vi "Mem_LvDataToMemory_NOPTR.vi"(8 "error in (no error)":errorcluster, 10 "Payload":variant) -> (0 "error out":errorcluster, 1 "Supported Type?":bool, 2 "ByteArray":u8[](array[numeric]))   [LabVIEW 2019, in "Memory Data Access.lvlib"]
uses:
  Memory Data Access.lvlib
  <vilib>/Utility/Data Type/Type Definitions/Data Type.ctl
  Global/Global.vi
  <vilib>/Utility/Data Type/NI_Data Type.lvlib
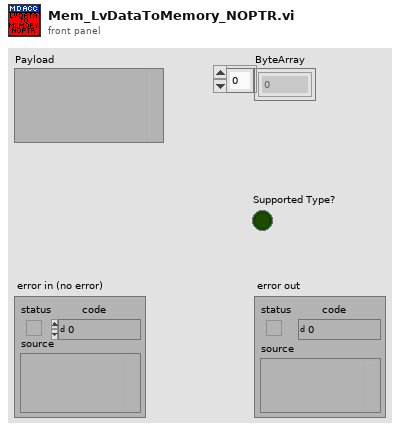
[diagram p1: front panel]
types:
  T1 = typedef "NI_Data Type.lvlib/Data Type.ctl" = enum8{"Invalid Type", "Void", "I8", "I16", "I32", "I64", "U8", "U16", "U32", "U64", "Single Float", "Double Float", "Extended Float", "Single Complex", "Double Complex", "Extended Complex", "Enum U8", "Enum U16", "Enum U32", "Enum U64", "Single Float With Unit", "Double Float With Unit", "Extended Float With Unit", "Single Complex with Unit", "Double Complex with Unit", "Extended Complex with Unit", "Boolean", "String", "Path", "Picture", "Tag", "Array", "Cluster", "Variant", "LV Variant", "Waveform", "Timestamp", "Digital Waveform", "Digital Data", "ExpressData", "Refnum", "External Data", "VI", "Poly VI", "LabVIEW Class Instance", "Fixed Point", "Set Collection", "Map Collection"}
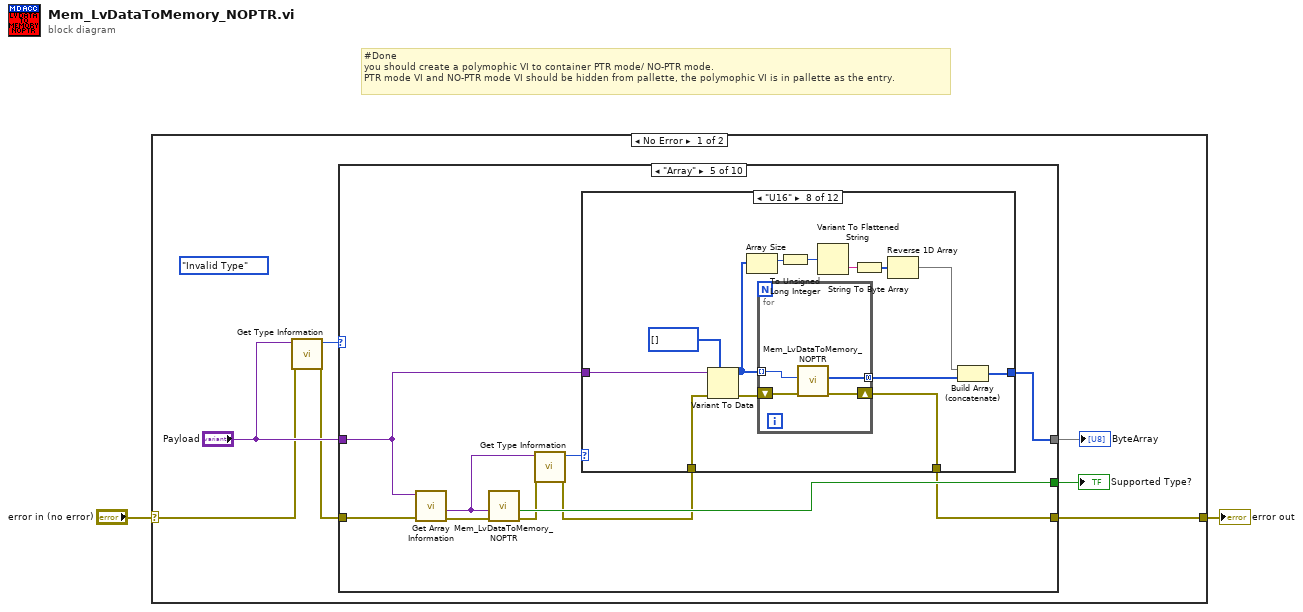
[diagram p0: block diagram]
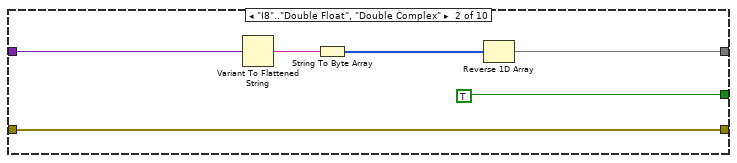
[diagram p3: hidden frame]
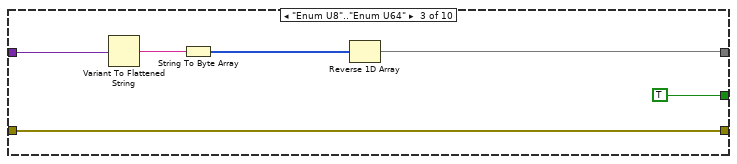
[diagram p4: hidden frame]
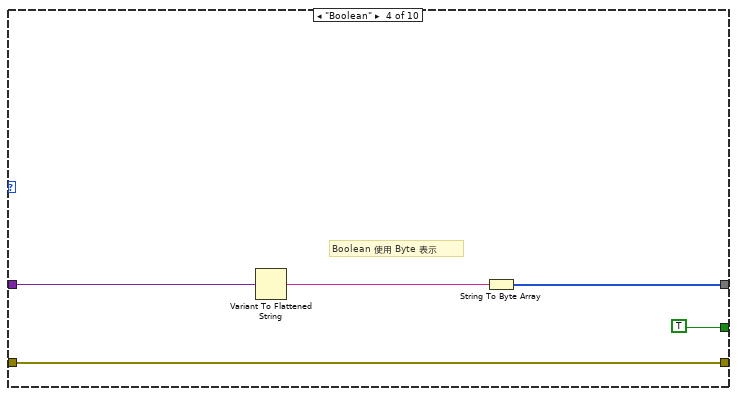
[diagram p5: hidden frame]
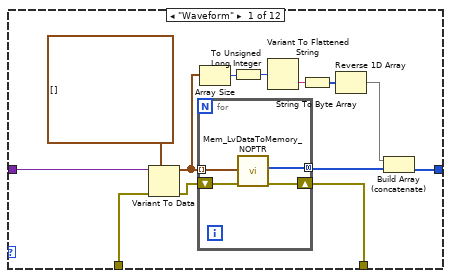
[diagram p6: hidden frame]
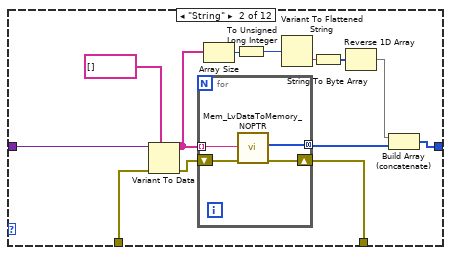
[diagram p7: hidden frame]
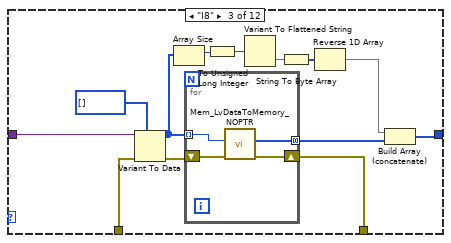
[diagram p8: hidden frame]
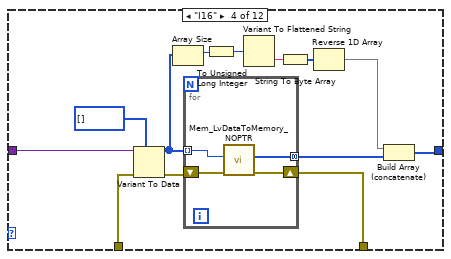
[diagram p9: hidden frame]
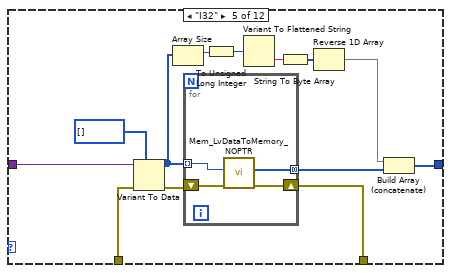
[diagram p10: hidden frame]
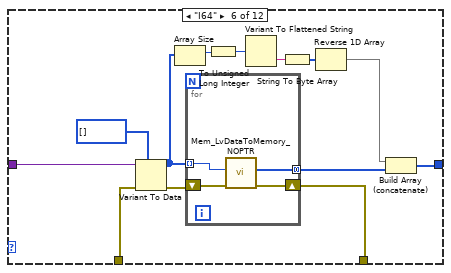
[diagram p11: hidden frame]
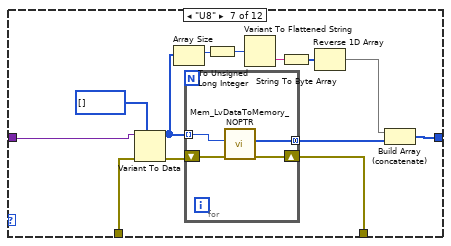
[diagram p12: hidden frame]
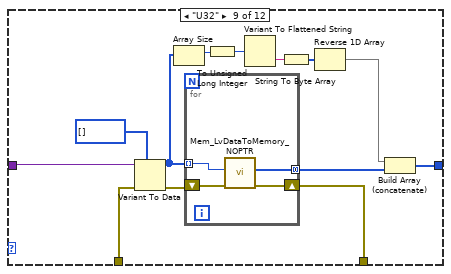
[diagram p13: hidden frame]
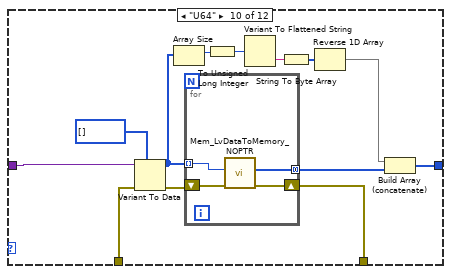
[diagram p14: hidden frame]
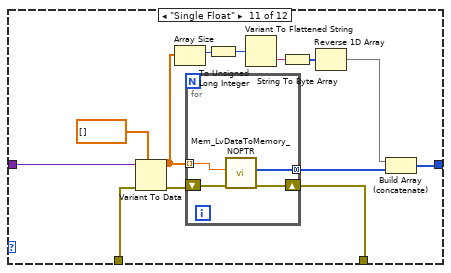
[diagram p15: hidden frame]
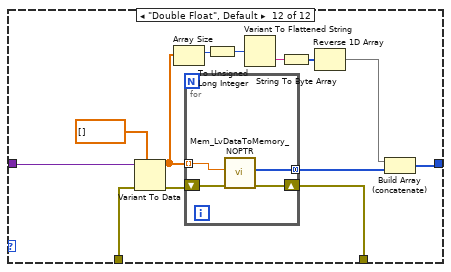
[diagram p16: hidden frame]
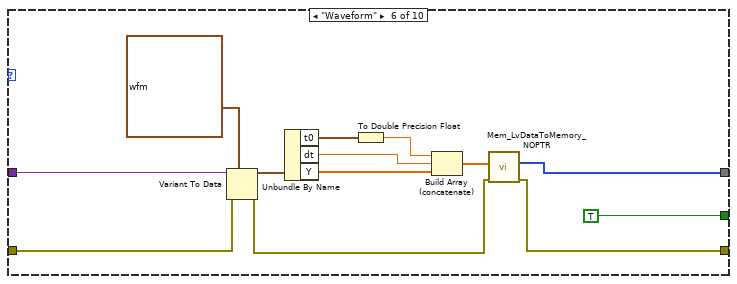
[diagram p17: hidden frame]
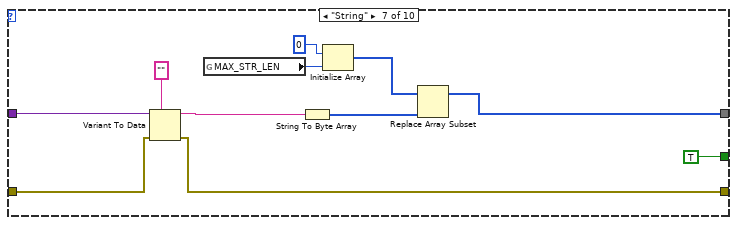
[diagram p18: hidden frame]
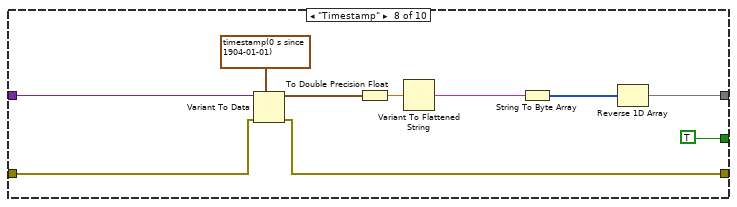
[diagram p19: hidden frame]
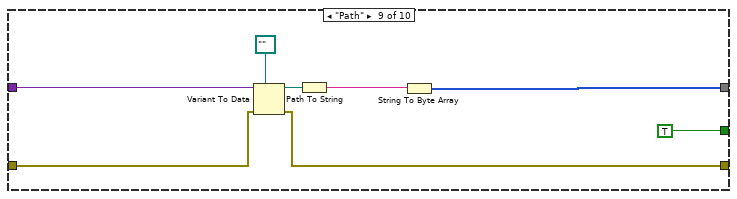
[diagram p20: hidden frame]
diagram:
  # "#Done\nyou should create a polymophic VI to container PTR mode/ NO-PTR mode.\nPTR mode VI and NO-PTR mode VI should be hidden from pallette, the polymophic VI is in pallette as the entry."
  n1 = case shown="No Error" "error in (no error)" {
    selector: "error in (no error)" -> [w4 w298]
    tunnel: [w9 w298] -> w2
    frame No Error {
      (unwired) Data_Type."Invalid Type" ("Type")
      n2 = call <vilib>:"Get Type Information.vi"("error in (no error)"=w4, "variant"="Payload") -> ("error out"=w3:errorcluster, "type"=w5:T1)  [unwired: 5 in, 3 out]
      n3 = case shown="\"Array\"" w5 {
        tunnel: w3 -> [w10 w16 w18 w27 w33 w246 w260 w270 w278 w284]
        tunnel: [w10 w16 w18 w27 w35 w243 w261 w271 w279 w285] -> w9
        tunnel: [_ w11 w19 w23 w37 w242 w263 w266 w281 w289] -> w8
        tunnel: "Payload" -> [_ w14 w21 w25 w34 w253 w264 w274 w282 w292]
        tunnel: [_ TRUE TRUE ("Supported Type?") TRUE w36 TRUE TRUE TRUE TRUE w287] -> w7
        frame "Invalid Type", Default {
        }
        frame "I8".."Double Float", "Double Complex" {
          n4 = Variant To Flattened String(Variant=w14) -> (data string=w13:string)  [unwired: 1 out]
          n5 = String To Byte Array(string=w13) -> (unsigned byte array=w12:u8[])
          n6 = Reverse 1D Array(array=w12) -> (reversed array=w11:u8[])
        }
        frame "Enum U8".."Enum U64" {
          n7 = Variant To Flattened String(Variant=w21) -> (data string=w22:string)  [unwired: 1 out]
          n8 = String To Byte Array(string=w22) -> (unsigned byte array=w20:u8[])
          n9 = Reverse 1D Array(array=w20) -> (reversed array=w19:u8[])
        }
        frame "Boolean" {
          # "Boolean 使用 Byte 表示"
          n10 = Variant To Flattened String(Variant=w25) -> (data string=w24:string)  [unwired: 1 out]
          n11 = String To Byte Array(string=w24) -> (unsigned byte array=w23:u8[])
        }
        frame "Array" {
          n12 = call <vilib>:"Get Array Information.vi"("error in (no error)"=w33, "variant"=w34) -> ("error out"=w32:errorcluster, "array element data type"=w30:variant)  [unwired: 6 in, 2 out]
          n13 = call "Mem_LvDataToMemory_NOPTR.vi"("error in (no error)"=w32, "Payload"=w30) -> ("error out"=w29:errorcluster, "Supported Type?"=w36:bool)  [unwired: 7 in, 1 out]
          n14 = call <vilib>:"Get Type Information.vi"("error in (no error)"=w29, "variant"=w30) -> ("error out"=w28:errorcluster, "type"=w31:T1)  [unwired: 5 in, 3 out]
          n15 = case shown="\"U16\"" w31 {
            tunnel: [w47 w64 w73 w90 w107 w124 w144 w161 w178 w195 w211 w226] -> w37
            tunnel: w34 -> [w50 w67 w83 w91 w110 w127 w143 w160 w177 w194 w212 w229]
            tunnel: w28 -> [w45 w62 w84 w93 w109 w126 w142 w159 w176 w193 w210 w228]
            tunnel: [w44 w61 w74 w92 w108 w125 w141 w158 w175 w192 w209 w227] -> w35
            frame "Waveform" {
              n16 = Variant To Data(error in=w45, type=waveform(dbl)[] [] ("Waveform"), Variant=w50) -> (data=w43:waveform(dbl)[], error out=w46:errorcluster)
              n17 = for {
                tunnel: w43 -> [w54] mode=indexing
                tunnel: [w53] -> w48 mode=concatenating
                shift-right: [w51] -> w44
                shift-left: w46 -> [w52]
                n18 = call "Mem_LvDataToMemory_NOPTR.vi"("error in (no error)"=w52, "Payload"=w54) -> ("error out"=w51:errorcluster, "ByteArray"=w53:u8[])  [unwired: 7 in, 1 out]
              }
              n19 = Array Size(array=w43) -> (size(s)=w42:i32)
              n20 = To Unsigned Long Integer(number=w42) -> (unsigned 32bit integer=w40:u32)
              n21 = Variant To Flattened String(Variant=w40) -> (data string=w41:string)  [unwired: 1 out]
              n22 = String To Byte Array(string=w41) -> (unsigned byte array=w39:u8[])
              n23 = Reverse 1D Array(array=w39) -> (reversed array=w38:u8[])
              n24 = Build Array (concatenate)(w38, w48) -> (w47:u8[])
            }
            frame "String" {
              n25 = Variant To Data(error in=w62, type=string[] [] ("Waveform"), Variant=w67) -> (data=w60:string[], error out=w63:errorcluster)
              n26 = for {
                tunnel: w60 -> [w71] mode=indexing
                tunnel: [w70] -> w65 mode=concatenating
                shift-right: [w68] -> w61
                shift-left: w63 -> [w69]
                n27 = call "Mem_LvDataToMemory_NOPTR.vi"("error in (no error)"=w69, "Payload"=w71) -> ("error out"=w68:errorcluster, "ByteArray"=w70:u8[])  [unwired: 7 in, 1 out]
              }
              n28 = Array Size(array=w60) -> (size(s)=w59:i32)
              n29 = To Unsigned Long Integer(number=w59) -> (unsigned 32bit integer=w57:u32)
              n30 = Variant To Flattened String(Variant=w57) -> (data string=w58:string)  [unwired: 1 out]
              n31 = String To Byte Array(string=w58) -> (unsigned byte array=w56:u8[])
              n32 = Reverse 1D Array(array=w56) -> (reversed array=w55:u8[])
              n33 = Build Array (concatenate)(w55, w65) -> (w64:u8[])
            }
            frame "I8" {
              n34 = Variant To Data(error in=w84, type=i8[] [], Variant=w83) -> (data=w72:i8[], error out=w82:errorcluster)
              n35 = Array Size(array=w72) -> (size(s)=w78:i32)
              n36 = for {
                tunnel: [w88] -> w75 mode=concatenating
                shift-right: [w86] -> w74
                shift-left: w82 -> [w87]
                tunnel: w72 -> [w85] mode=indexing
                n37 = call "Mem_LvDataToMemory_NOPTR.vi"("error in (no error)"=w87, "Payload"=w85) -> ("error out"=w86:errorcluster, "ByteArray"=w88:u8[])  [unwired: 7 in, 1 out]
              }
              n38 = To Unsigned Long Integer(number=w78) -> (unsigned 32bit integer=w79:u32)
              n39 = Variant To Flattened String(Variant=w79) -> (data string=w80:string)  [unwired: 1 out]
              n40 = String To Byte Array(string=w80) -> (unsigned byte array=w77:u8[])
              n41 = Reverse 1D Array(array=w77) -> (reversed array=w76:u8[])
              n42 = Build Array (concatenate)(w76, w75) -> (w73:u8[])
            }
            frame "I16" {
              n43 = Variant To Data(error in=w93, type=i16[] [], Variant=w91) -> (data=w89:i16[], error out=w101:errorcluster)
              n44 = Array Size(array=w89) -> (size(s)=w97:i32)
              n45 = for {
                tunnel: [w105] -> w94 mode=concatenating
                shift-right: [w103] -> w92
                shift-left: w101 -> [w104]
                tunnel: w89 -> [w102] mode=indexing
                n46 = call "Mem_LvDataToMemory_NOPTR.vi"("error in (no error)"=w104, "Payload"=w102) -> ("error out"=w103:errorcluster, "ByteArray"=w105:u8[])  [unwired: 7 in, 1 out]
              }
              n47 = To Unsigned Long Integer(number=w97) -> (unsigned 32bit integer=w98:u32)
              n48 = Variant To Flattened String(Variant=w98) -> (data string=w99:string)  [unwired: 1 out]
              n49 = String To Byte Array(string=w99) -> (unsigned byte array=w96:u8[])
              n50 = Reverse 1D Array(array=w96) -> (reversed array=w95:u8[])
              n51 = Build Array (concatenate)(w95, w94) -> (w90:u8[])
            }
            frame "I32" {
              n52 = Variant To Data(error in=w109, type=i32[] [], Variant=w110) -> (data=w106:i32[], error out=w118:errorcluster)
              n53 = Array Size(array=w106) -> (size(s)=w114:i32)
              n54 = for {
                tunnel: [w122] -> w111 mode=concatenating
                shift-right: [w120] -> w108
                shift-left: w118 -> [w121]
                tunnel: w106 -> [w119] mode=indexing
                n55 = call "Mem_LvDataToMemory_NOPTR.vi"("error in (no error)"=w121, "Payload"=w119) -> ("error out"=w120:errorcluster, "ByteArray"=w122:u8[])  [unwired: 7 in, 1 out]
              }
              n56 = To Unsigned Long Integer(number=w114) -> (unsigned 32bit integer=w115:u32)
              n57 = Variant To Flattened String(Variant=w115) -> (data string=w116:string)  [unwired: 1 out]
              n58 = String To Byte Array(string=w116) -> (unsigned byte array=w113:u8[])
              n59 = Reverse 1D Array(array=w113) -> (reversed array=w112:u8[])
              n60 = Build Array (concatenate)(w112, w111) -> (w107:u8[])
            }
            frame "I64" {
              n61 = Variant To Data(error in=w126, type=i64[] [], Variant=w127) -> (data=w123:i64[], error out=w135:errorcluster)
              n62 = Array Size(array=w123) -> (size(s)=w131:i32)
              n63 = for {
                tunnel: [w139] -> w128 mode=concatenating
                shift-right: [w137] -> w125
                shift-left: w135 -> [w138]
                tunnel: w123 -> [w136] mode=indexing
                n64 = call "Mem_LvDataToMemory_NOPTR.vi"("error in (no error)"=w138, "Payload"=w136) -> ("error out"=w137:errorcluster, "ByteArray"=w139:u8[])  [unwired: 7 in, 1 out]
              }
              n65 = To Unsigned Long Integer(number=w131) -> (unsigned 32bit integer=w132:u32)
              n66 = Variant To Flattened String(Variant=w132) -> (data string=w133:string)  [unwired: 1 out]
              n67 = String To Byte Array(string=w133) -> (unsigned byte array=w130:u8[])
              n68 = Reverse 1D Array(array=w130) -> (reversed array=w129:u8[])
              n69 = Build Array (concatenate)(w129, w128) -> (w124:u8[])
            }
            frame "U8" {
              n70 = Variant To Data(error in=w142, type=u8[] [], Variant=w143) -> (data=w140:u8[], error out=w152:errorcluster)
              n71 = Array Size(array=w140) -> (size(s)=w148:i32)
              n72 = for {
                tunnel: [w156] -> w145 mode=concatenating
                shift-right: [w154] -> w141
                shift-left: w152 -> [w155]
                tunnel: w140 -> [w153] mode=indexing
                n73 = call "Mem_LvDataToMemory_NOPTR.vi"("error in (no error)"=w155, "Payload"=w153) -> ("error out"=w154:errorcluster, "ByteArray"=w156:u8[])  [unwired: 7 in, 1 out]
              }
              n74 = To Unsigned Long Integer(number=w148) -> (unsigned 32bit integer=w149:u32)
              n75 = Variant To Flattened String(Variant=w149) -> (data string=w150:string)  [unwired: 1 out]
              n76 = String To Byte Array(string=w150) -> (unsigned byte array=w147:u8[])
              n77 = Reverse 1D Array(array=w147) -> (reversed array=w146:u8[])
              n78 = Build Array (concatenate)(w146, w145) -> (w144:u8[])
            }
            frame "U16" {
              n79 = Variant To Data(error in=w159, type=u16[] [], Variant=w160) -> (data=w157:u16[], error out=w169:errorcluster)
              n80 = Array Size(array=w157) -> (size(s)=w165:i32)
              n81 = for {
                tunnel: [w173] -> w162 mode=concatenating
                shift-right: [w171] -> w158
                shift-left: w169 -> [w172]
                tunnel: w157 -> [w170] mode=indexing
                n82 = call "Mem_LvDataToMemory_NOPTR.vi"("error in (no error)"=w172, "Payload"=w170) -> ("error out"=w171:errorcluster, "ByteArray"=w173:u8[])  [unwired: 7 in, 1 out]
              }
              n83 = To Unsigned Long Integer(number=w165) -> (unsigned 32bit integer=w166:u32)
              n84 = Variant To Flattened String(Variant=w166) -> (data string=w167:string)  [unwired: 1 out]
              n85 = String To Byte Array(string=w167) -> (unsigned byte array=w164:u8[])
              n86 = Reverse 1D Array(array=w164) -> (reversed array=w163:u8[])
              n87 = Build Array (concatenate)(w163, w162) -> (w161:u8[])
            }
            frame "U32" {
              n88 = Variant To Data(error in=w176, type=u32[] [], Variant=w177) -> (data=w174:u32[], error out=w186:errorcluster)
              n89 = Array Size(array=w174) -> (size(s)=w182:i32)
              n90 = for {
                tunnel: [w190] -> w179 mode=concatenating
                shift-right: [w188] -> w175
                shift-left: w186 -> [w189]
                tunnel: w174 -> [w187] mode=indexing
                n91 = call "Mem_LvDataToMemory_NOPTR.vi"("error in (no error)"=w189, "Payload"=w187) -> ("error out"=w188:errorcluster, "ByteArray"=w190:u8[])  [unwired: 7 in, 1 out]
              }
              n92 = To Unsigned Long Integer(number=w182) -> (unsigned 32bit integer=w183:u32)
              n93 = Variant To Flattened String(Variant=w183) -> (data string=w184:string)  [unwired: 1 out]
              n94 = String To Byte Array(string=w184) -> (unsigned byte array=w181:u8[])
              n95 = Reverse 1D Array(array=w181) -> (reversed array=w180:u8[])
              n96 = Build Array (concatenate)(w180, w179) -> (w178:u8[])
            }
            frame "U64" {
              n97 = Variant To Data(error in=w193, type=u64[] [], Variant=w194) -> (data=w191:u64[], error out=w203:errorcluster)
              n98 = Array Size(array=w191) -> (size(s)=w199:i32)
              n99 = for {
                tunnel: [w207] -> w196 mode=concatenating
                shift-right: [w205] -> w192
                shift-left: w203 -> [w206]
                tunnel: w191 -> [w204] mode=indexing
                n100 = call "Mem_LvDataToMemory_NOPTR.vi"("error in (no error)"=w206, "Payload"=w204) -> ("error out"=w205:errorcluster, "ByteArray"=w207:u8[])  [unwired: 7 in, 1 out]
              }
              n101 = To Unsigned Long Integer(number=w199) -> (unsigned 32bit integer=w200:u32)
              n102 = Variant To Flattened String(Variant=w200) -> (data string=w201:string)  [unwired: 1 out]
              n103 = String To Byte Array(string=w201) -> (unsigned byte array=w198:u8[])
              n104 = Reverse 1D Array(array=w198) -> (reversed array=w197:u8[])
              n105 = Build Array (concatenate)(w197, w196) -> (w195:u8[])
            }
            frame "Single Float" {
              n106 = Variant To Data(error in=w210, type=sgl[] [], Variant=w212) -> (data=w208:sgl[], error out=w220:errorcluster)
              n107 = Array Size(array=w208) -> (size(s)=w216:i32)
              n108 = for {
                tunnel: [w224] -> w213 mode=concatenating
                shift-right: [w222] -> w209
                shift-left: w220 -> [w223]
                tunnel: w208 -> [w221] mode=indexing
                n109 = call "Mem_LvDataToMemory_NOPTR.vi"("error in (no error)"=w223, "Payload"=w221) -> ("error out"=w222:errorcluster, "ByteArray"=w224:u8[])  [unwired: 7 in, 1 out]
              }
              n110 = To Unsigned Long Integer(number=w216) -> (unsigned 32bit integer=w217:u32)
              n111 = Variant To Flattened String(Variant=w217) -> (data string=w218:string)  [unwired: 1 out]
              n112 = String To Byte Array(string=w218) -> (unsigned byte array=w215:u8[])
              n113 = Reverse 1D Array(array=w215) -> (reversed array=w214:u8[])
              n114 = Build Array (concatenate)(w214, w213) -> (w211:u8[])
            }
            frame "Double Float", Default {
              n115 = Variant To Data(error in=w228, type=dbl[] [], Variant=w229) -> (data=w225:dbl[], error out=w237:errorcluster)
              n116 = Array Size(array=w225) -> (size(s)=w233:i32)
              n117 = for {
                tunnel: [w241] -> w230 mode=concatenating
                shift-right: [w239] -> w227
                shift-left: w237 -> [w240]
                tunnel: w225 -> [w238] mode=indexing
                n118 = call "Mem_LvDataToMemory_NOPTR.vi"("error in (no error)"=w240, "Payload"=w238) -> ("error out"=w239:errorcluster, "ByteArray"=w241:u8[])  [unwired: 7 in, 1 out]
              }
              n119 = To Unsigned Long Integer(number=w233) -> (unsigned 32bit integer=w234:u32)
              n120 = Variant To Flattened String(Variant=w234) -> (data string=w235:string)  [unwired: 1 out]
              n121 = String To Byte Array(string=w235) -> (unsigned byte array=w232:u8[])
              n122 = Reverse 1D Array(array=w232) -> (reversed array=w231:u8[])
              n123 = Build Array (concatenate)(w231, w230) -> (w226:u8[])
            }
          }
        }
        frame "Waveform" {
          n124 = Variant To Data(error in=w246, type=waveform(dbl) {"t0"=timestamp(0 s since 1904-01-01), "dt"=1.0, "Y"=[]} ("Waveform"), Variant=w253) -> (data=w251:waveform(dbl), error out=w244:errorcluster)
          n125 = Unbundle By Name(w251) -> ("t0"=w249:timestamp, "dt"=w247:dbl, "Y"=w250:dbl[])
          n126 = To Double Precision Float(number=w249) -> (double precision float=w248:dbl)
          n127 = Build Array (concatenate)(w248, w247, w250) -> (w245:dbl[])
          n128 = call "Mem_LvDataToMemory_NOPTR.vi"("error in (no error)"=w244, "Payload"=w245) -> ("error out"=w243:errorcluster, "ByteArray"=w242:u8[])  [unwired: 7 in, 1 out]
        }
        frame "String" {
          n129 = Variant To Data(error in=w260, type="" ("Waveform"), Variant=w264) -> (data=w259:string, error out=w261:errorcluster)
          n130 = global read "Global.vi" "MAX_STR_LEN"() -> (w255:u32)
          n131 = String To Byte Array(string=w259) -> (unsigned byte array=w256:u8[])
          n132 = Initialize Array(u8 0 ("*(type *) &x"), w255) -> (w257:u8[])
          n133 = Replace Array Subset(array=w257, new element=w256) -> (w263:u8[])  [unwired: 1 in]
        }
        frame "Timestamp" {
          n134 = Variant To Data(error in=w270, type=timestamp(0 s since 1904-01-01) ("Waveform"), Variant=w274) -> (data=w269:timestamp, error out=w271:errorcluster)
          n135 = To Double Precision Float(number=w269) -> (double precision float=w268:dbl)
          n136 = Variant To Flattened String(Variant=w268) -> (data string=w273:string)  [unwired: 1 out]
          n137 = String To Byte Array(string=w273) -> (unsigned byte array=w267:u8[])
          n138 = Reverse 1D Array(array=w267) -> (reversed array=w266:u8[])
        }
        frame "Path" {
          n139 = Variant To Data(error in=w278, type=path "" ("Waveform"), Variant=w282) -> (data=w277:path, error out=w279:errorcluster)
          n140 = Path To String(path=w277) -> (string=w276:string)
          n141 = String To Byte Array(string=w276) -> (unsigned byte array=w281:u8[])
        }
        frame "Cluster" {
          n142 = call <userlib>:"Cluster to Array of VData__ogtk.vi"("error in (no error)"=w284, "Cluster"=w292) -> ("error out"=w286:errorcluster, "Array of VData"=w291:variant[])  [unwired: 8 in]
          n143 = for {
            tunnel: w291 -> [w297] mode=indexing
            tunnel: [w296] -> w290 mode=concatenating
            tunnel: [w295] -> w288 mode=indexing
            shift-right: [w293] -> w285
            shift-left: w286 -> [w294]
            n144 = call "Mem_LvDataToMemory_NOPTR.vi"("error in (no error)"=w294, "Payload"=w297) -> ("error out"=w293:errorcluster, "Supported Type?"=w295:bool, "ByteArray"=w296:u8[])  [unwired: 7 in]
          }
          n145 = Build Array (concatenate)(w290) -> (w289:u8[])
          n146 = And Array Elements(Boolean array=w288) -> (logical AND=w287:bool)
        }
      }
      "ByteArray" <- w8
      "Supported Type?" <- w7
    }
    frame Error {
    }
  }
  "error out" <- w2
